vi "Get_Access_Scope.vi"(8 "error in (no error)":errorcluster, 11 "AB_Source_VI in":refnum<class "AB_Source_VI.lvclass">) -> (0 "error out":errorcluster, 2 "Source Scope":T1(ring), 3 "AB_Source_VI out":refnum<class "AB_Source_VI.lvclass">)   [LabVIEW 2020, in "AB_Source_VI.lvclass"]
uses:
  <vilib>/AppBuilder/AB_Classes/Source/VI/AB_Source_VI.lvclass
  <vilib>/AppBuilder/AB_Classes/Source/VI/AB_Source_VI.lvclass/AB_Source_VI.ctl
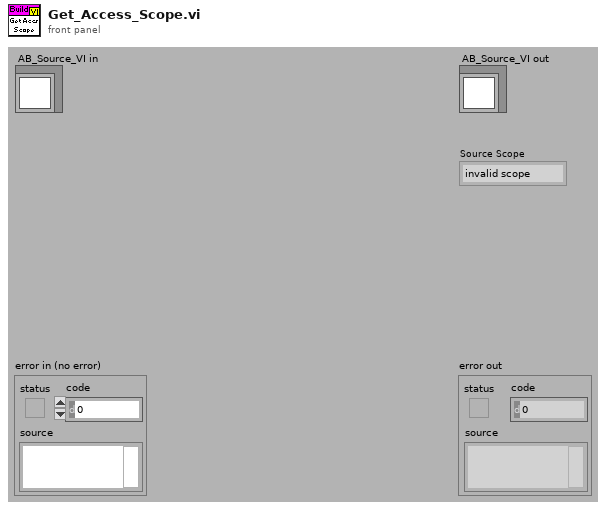
[diagram p1: front panel]
types:
  T1 = enum32{"invalid scope", "public", "private", "protected", "community"}
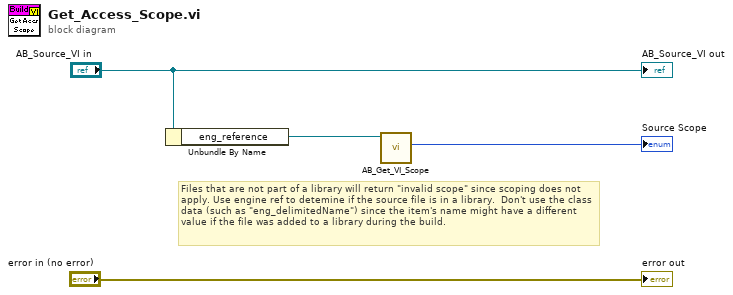
[diagram p0: block diagram]
diagram:
  # "Files that are not part of a library will return \"invalid scope\" since scoping does not apply. Use engine ref to detemine if the source file is in a library.  Don't use the class data (such as \"eng_delimitedName\") since the item's name might have a different value if the file was added to a library during the build."
  n1 = Unbundle By Name("AB_Source_VI in") -> ("eng_reference"=w2:refnum<vi>)
  n2 = call <vilib>:"AB_Get_VI_Scope.vi"("vi reference"=w2) -> ("Source Scope"=→"Source Scope":T1)  [unwired: 8 in, 2 out]
  "error out" <- "error in (no error)"
  "AB_Source_VI out" <- "AB_Source_VI in"
